vi "getAvailableShiftSpeeds.vi"(8 "error in (no error)":errorcluster, 11 "AndorIKonAcquisitor.lvclass in":refnum<class "AndorIKonAcquisitor.lvclass">) -> (0 "error out":errorcluster, 2 "Available Shift Speeds":T1={"Vertical Shift Speeds"=[0.5250000357627869, 0.875, 1.5750000476837158, 2.9749999046325684, 5.775000095367432, 11.375, 22.57499885559082, 44.97500228881836], "Horizontal Shift Speeds"=[0.05, 1.0, 2.5]} {"Horizontal Shift Speeds" format="%#_9g"; "Vertical Shift Speeds" format="%#_9g"}, 3 "AndorIKonAcquisitor.lvclass out":refnum<class "AndorIKonAcquisitor.lvclass">)   [LabVIEW 2009, in "Hardware.lvlib" / "Channels.lvlib" / "AndorIKonAcquisitor.lvclass"]
uses:
  AndorIKonAcquisitor.lvclass
  AndorIKonAcquisitor.lvclass/AndorIKonAcquisitor.ctl
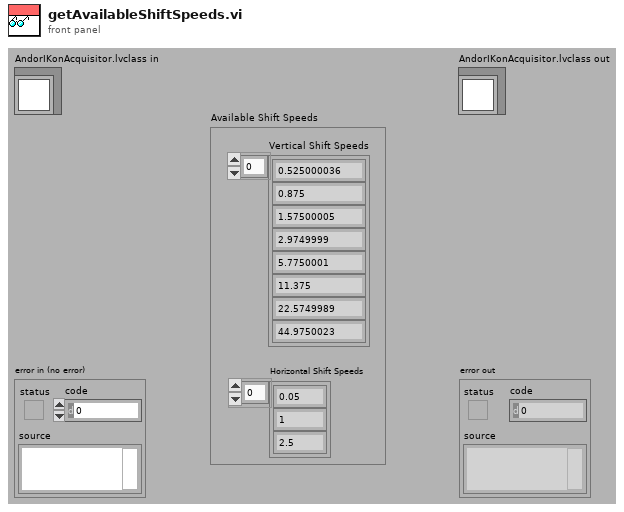
[diagram p1: front panel]
types:
  T1 = cluster{"Vertical Shift Speeds":dbl[], "Horizontal Shift Speeds":dbl[]}
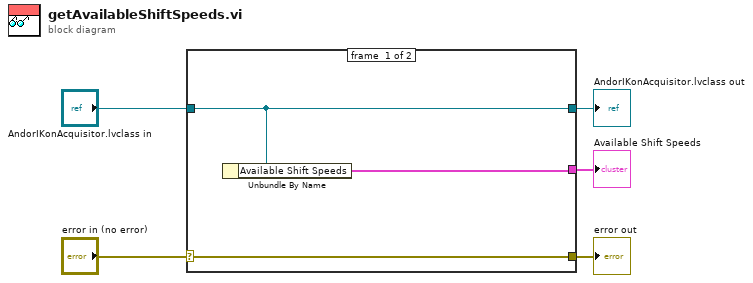
[diagram p0: block diagram]
diagram:
  n1 = case shown="No Error" "error in (no error)" {
    selector: "error in (no error)" -> [w8 w9]
    tunnel: [w8 w9] -> w4
    tunnel: [w7 w10] -> w2
    tunnel: "AndorIKonAcquisitor.lvclass in" -> [w7 w10]
    tunnel: [w6 _] -> w1
    frame #0 {
      n2 = Unbundle By Name(w7) -> ("Available Shift Speeds"=w6:T1)
    }
    frame #1 {
    }
  }
  "error out" <- w4
  "AndorIKonAcquisitor.lvclass out" <- w2
  "Available Shift Speeds" <- w1
